vi "Type of a Substring.VI"(1 "item":string) -> (0 "type":i32)   [LabVIEW 2017, in "NI_Gmath.lvlib"]
uses:
  <vilib>/gmath/NI_Gmath.lvlib
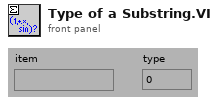
[diagram p1: front panel]
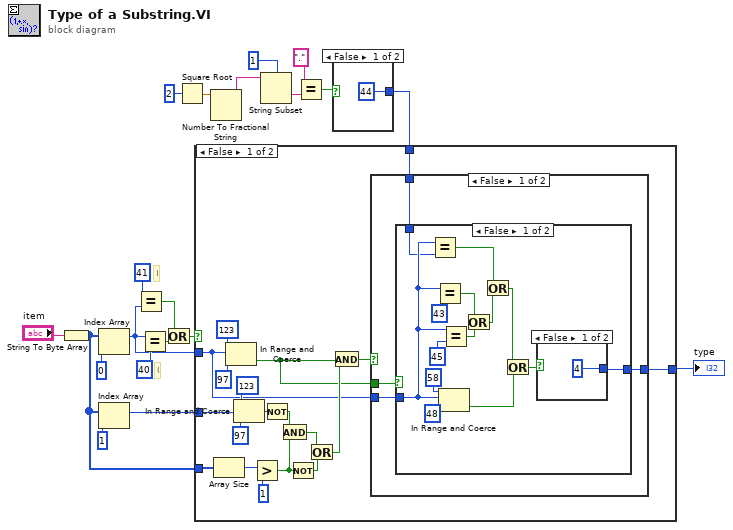
[diagram p0: block diagram]
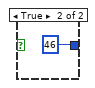
[diagram p2: hidden frame]
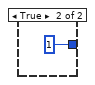
[diagram p3: hidden frame]
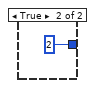
[diagram p4: hidden frame]
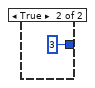
[diagram p5: hidden frame]
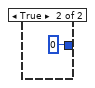
[diagram p6: hidden frame]
diagram:
  w7 = 1
  # ")"
  # "("
  n1 = String To Byte Array(string="item") -> (unsigned byte array=w10:u8[])
  n2 = Index Array(array=w10, index=0) -> (element=w15:u8)
  n3 = Index Array(array=w10, index=1) -> (element=w9:u8)
  n4 = Equal?(x=41, y=w15) -> (x = y?=w13:bool)
  n5 = Equal?(x=w15, y=40) -> (x = y?=w14:bool)
  n6 = Or(x=w13, y=w14) -> (x .or. y?=w12:bool)
  n7 = Square Root(x=2) -> (sqrt(x)=w5:dbl)
  n8 = Number To Fractional String(number=w5) -> (F-format string=w8:string)  [unwired: 3 in]
  n9 = String Subset(string=w8, offset (0)=w7, length (rest)=w7) -> (substring=w4:string)
  n10 = Equal?(x=".", y=w4) -> (x = y?=w2:bool)
  n11 = case shown="False" w2 {
    tunnel: [44 46] -> w1
    frame False {
    }
    frame True {
    }
  }
  n12 = case shown="False" w12 {
    tunnel: w15 -> [w26 _]
    tunnel: [w41 0] -> w17
    tunnel: w10 -> [w38 _]
    tunnel: w9 -> [w25 _]
    tunnel: w1 -> [w23 _]
    frame False {
      n13 = Array Size(array=w38) -> (size(s)=w37:i32)
      n14 = In Range and Coerce(upper limit=123, x=w26, lower limit=97) -> (In Range?=w27:bool)  [unwired: 1 out]
      n15 = In Range and Coerce(upper limit=123, x=w25, lower limit=97) -> (In Range?=w33:bool)  [unwired: 1 out]
      n16 = Greater?(x=w37, y=1) -> (0:w32:bool)
      n17 = Not(x=w33) -> (.not. x?=w24:bool)
      n18 = And(x=w24, y=w32) -> (x .and. y?=w31:bool)
      n19 = Not(x=w32) -> (.not. x?=w30:bool)
      n20 = Or(x=w31, y=w30) -> (x .or. y?=w29:bool)
      n21 = And(x=w27, y=w29) -> (x .and. y?=w28:bool)
      n22 = case shown="False" w28 {
        tunnel: [w45 3] -> w41
        tunnel: w27 -> [w44 _]
        tunnel: w26 -> [w43 _]
        tunnel: w23 -> [w42 _]
        frame False {
          n23 = case shown="False" w44 {
            tunnel: w43 -> [w53 _]
            tunnel: [w47 2] -> w45
            tunnel: w42 -> [w46 _]
            frame False {
              n24 = Equal?(x=w53, y=w46) -> (x = y?=w52:bool)
              n25 = Equal?(x=w53, y=43) -> (x = y?=w54:bool)
              n26 = In Range and Coerce(upper limit=58, x=w53, lower limit=48) -> (In Range?=w50:bool)  [unwired: 1 out]
              n27 = Equal?(x=w53, y=45) -> (x = y?=w55:bool)
              n28 = Or(x=w54, y=w55) -> (x .or. y?=w51:bool)
              n29 = Or(x=w52, y=w51) -> (x .or. y?=w49:bool)
              n30 = Or(x=w49, y=w50) -> (x .or. y?=w48:bool)
              n31 = case shown="False" w48 {
                tunnel: [4 1] -> w47
                frame False {
                }
                frame True {
                }
              }
            }
            frame True {
            }
          }
        }
        frame True {
        }
      }
    }
    frame True {
    }
  }
  "type" <- w17
